vi "GetPoint.vi"(3 "error in":errorcluster, 5 "Image 2":T1(plugin-control)) -> (0 "error out":errorcluster, 1 "Y":sgl, 2 "X":sgl)   [LabVIEW 2011]
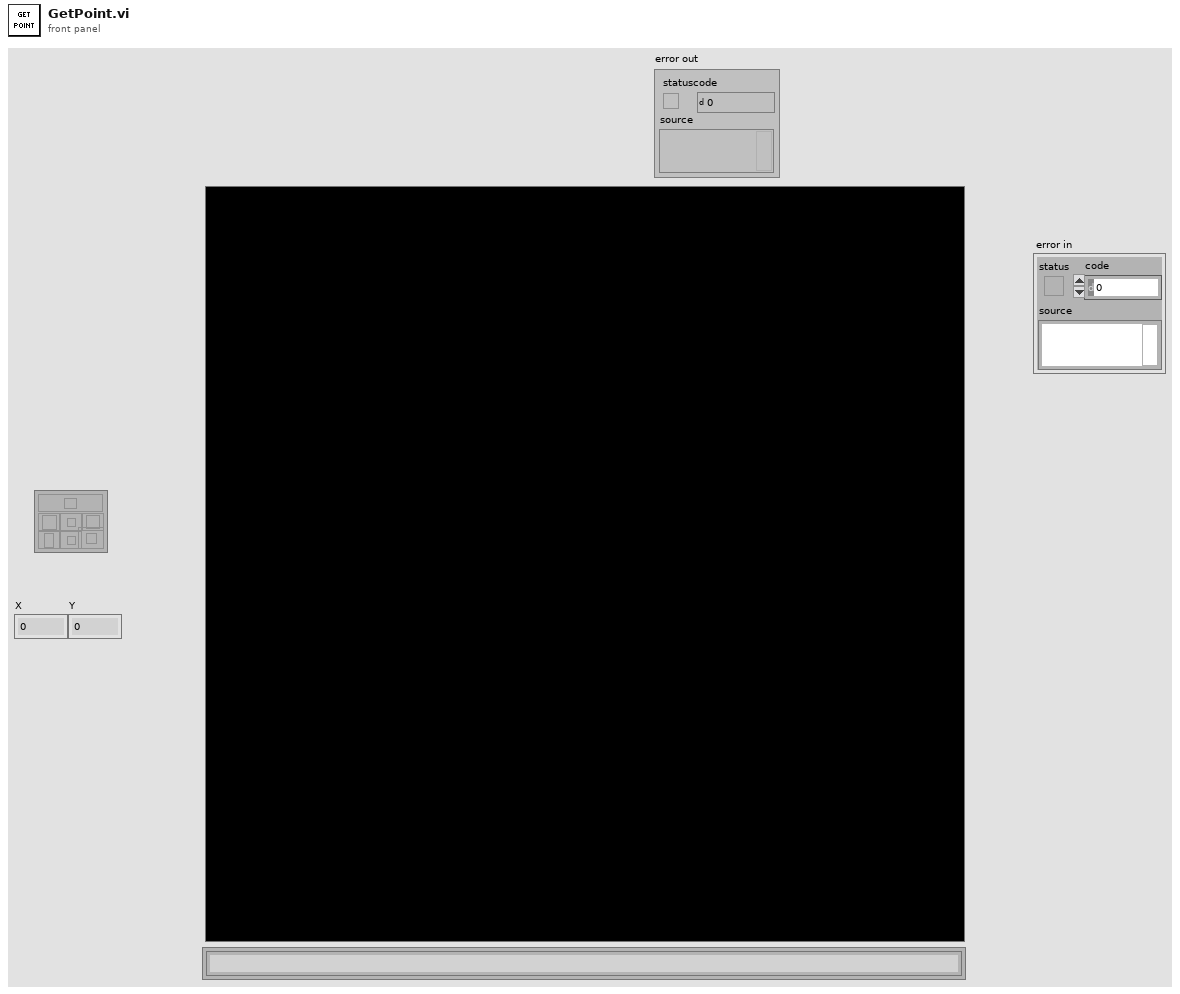
[diagram p1: front panel]
types:
  T1 = typedef "IMAQ Image.ctl" = refnum<image>
  T2 = typedef "IMAQ Point" = cluster{"X":sgl, "Y":sgl}
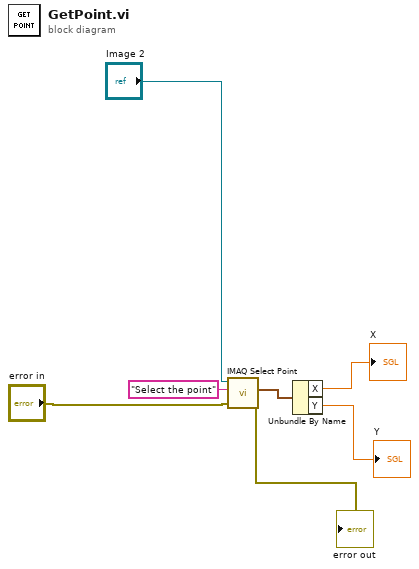
[diagram p0: block diagram]
diagram:
  n1 = call "IMAQ Select Point"("error in (no error)"="error in", "Prompt"="Select the point", "Image In"="Image 2") -> ("error out"=→"error out":errorcluster, "Point"=w5:T2)  [unwired: 5 in, 2 out]
  n2 = Unbundle By Name(w5) -> ("X"=→"X":sgl, "Y"=→"Y":sgl)
